vi "Jaccard assignemnts.vi"(9 "cluster centers in":string[](array[string])=["0 -1 1 -4 0 -4 1 -1 0", "0 -1 2 -2 0 -2 2 -1 0", "0 -2 3 -3 0 -3 3 -2 0", "0 -3 4 -4 0 -4 4 -3 0", "0 -1 1 -4 4 -3 0 -3 4 -4 1 -1 0", "0 -1 2 -2 3 -3 0 -3 3 -2 2 -1 0", "0 -4 1 -1 2 -2 0 -2 2 -1 1 -4 0", "0 -4 4 -3 3 -2 0 -2 3 -3 4 -4 0", "0 -1 1 -4 0 -2 3 -3 0 -3 3 -2 0 -4 1 -1 0", "0 -1 2 -2 0 -4 4 -3 0 -3 4 -4 0 -2 2 -1 0"], 11 "patterns in":string[](array[string])) -> (0 "distance values out enhanced multiset)":dbl[][](array[numeric]), 1 "distance values out (multiset)":dbl[][](array[numeric]), 2 "distance values out enhanced (set)":dbl[][](array[numeric]), 3 "distance values out (set)":dbl[][](array[numeric]))   [LabVIEW 2014]
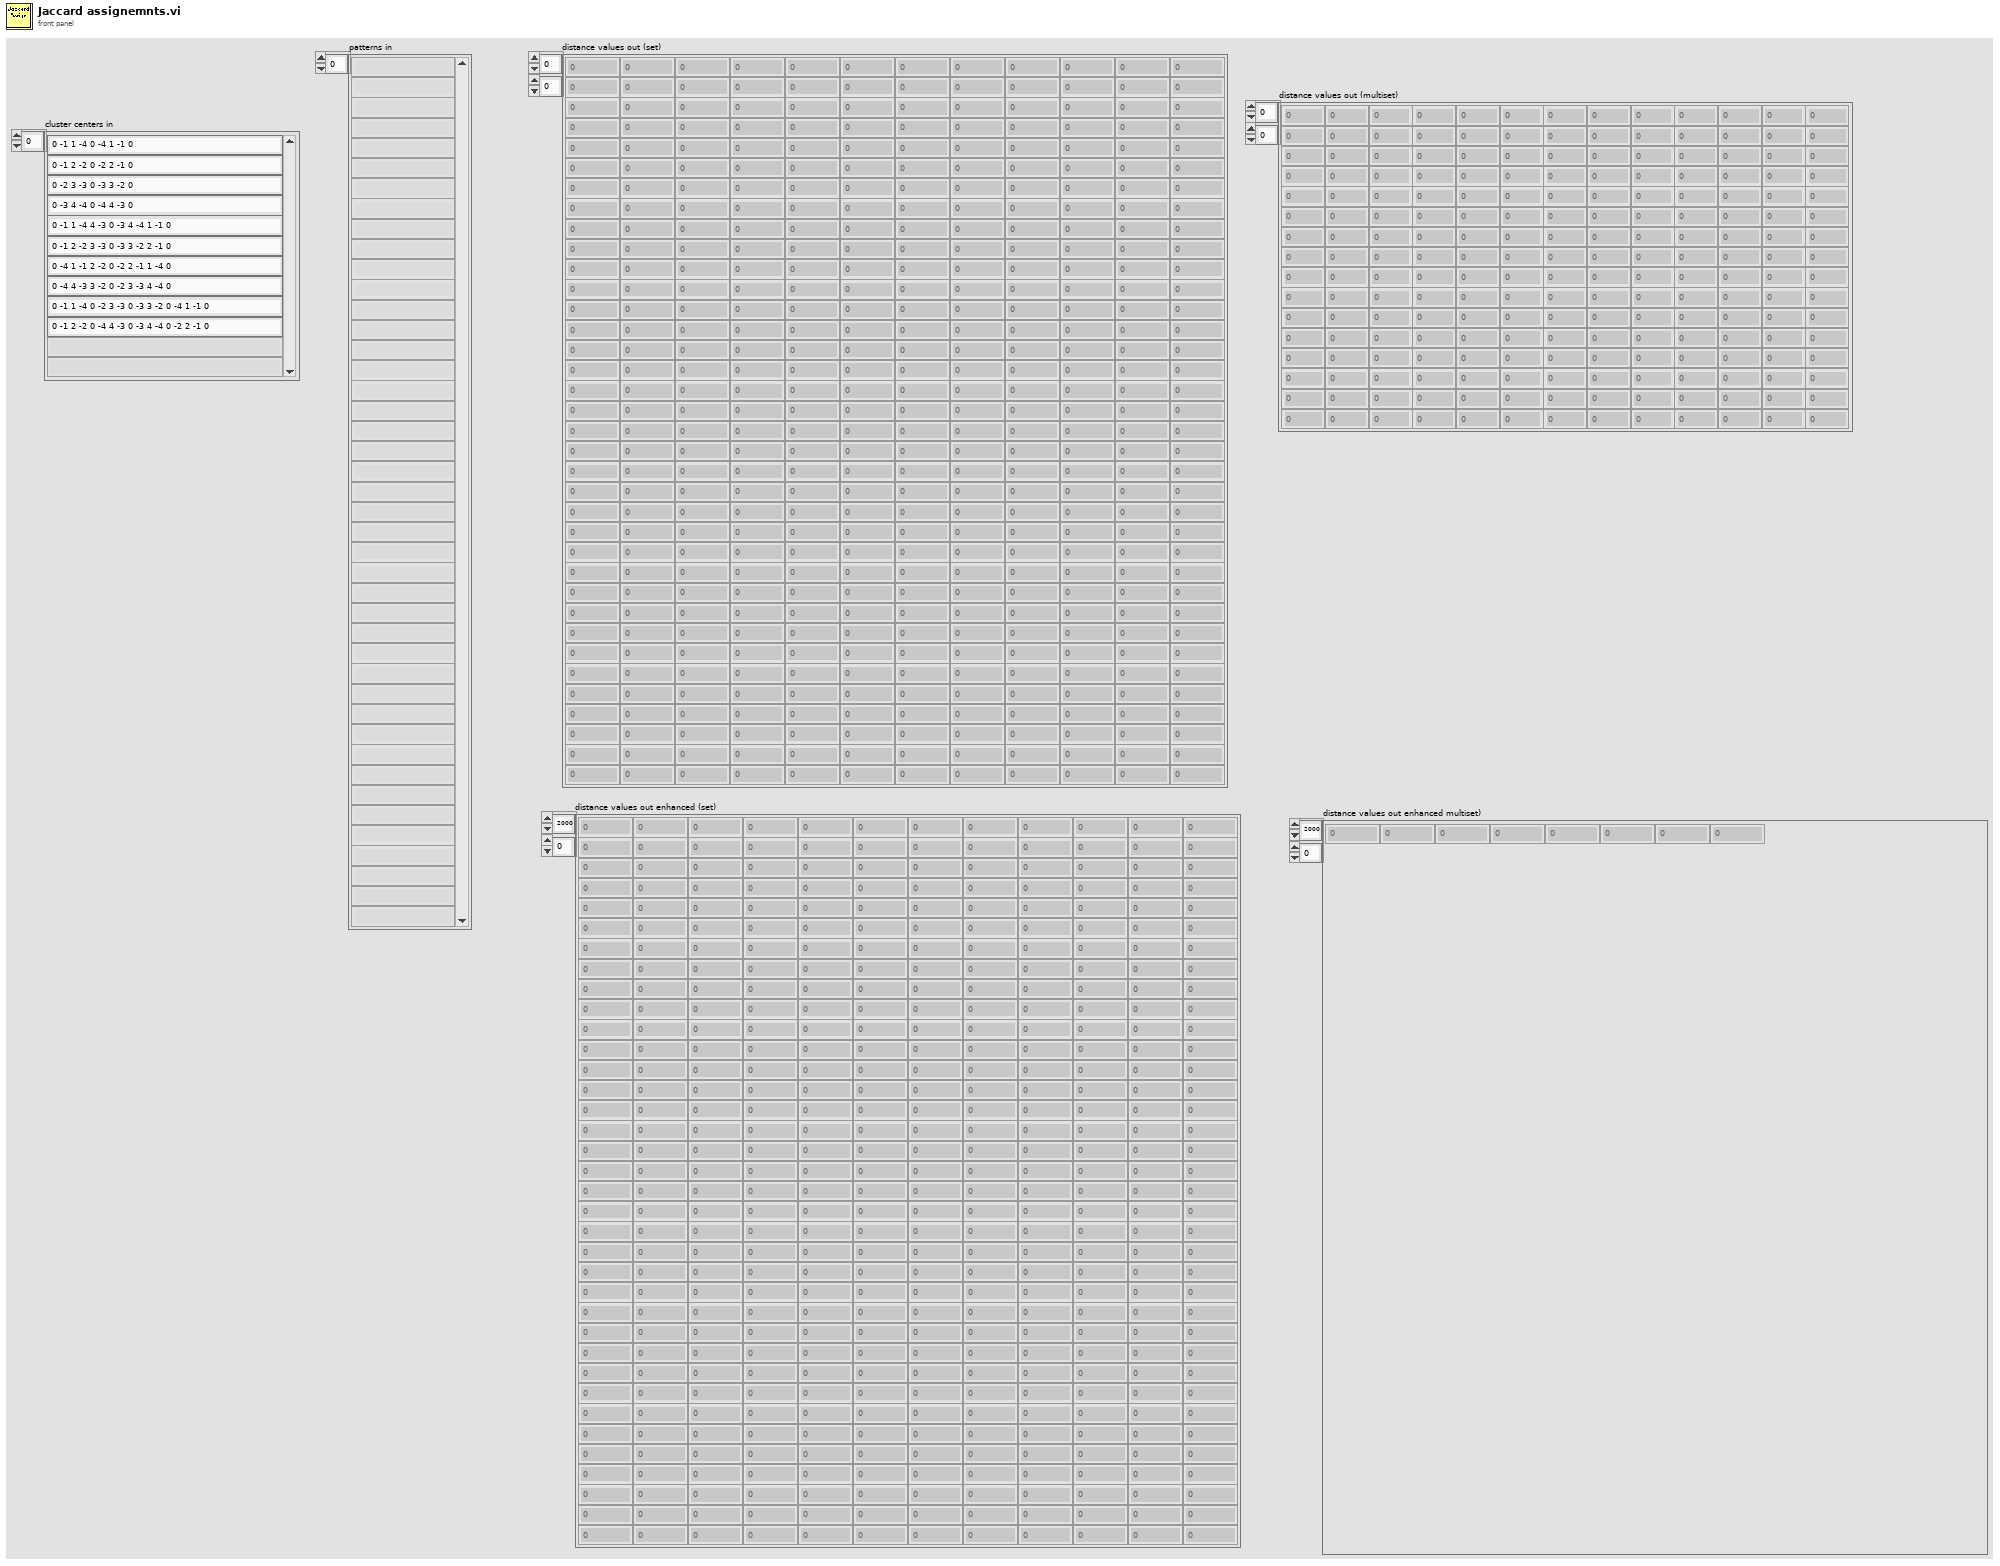
[diagram p1: front panel]
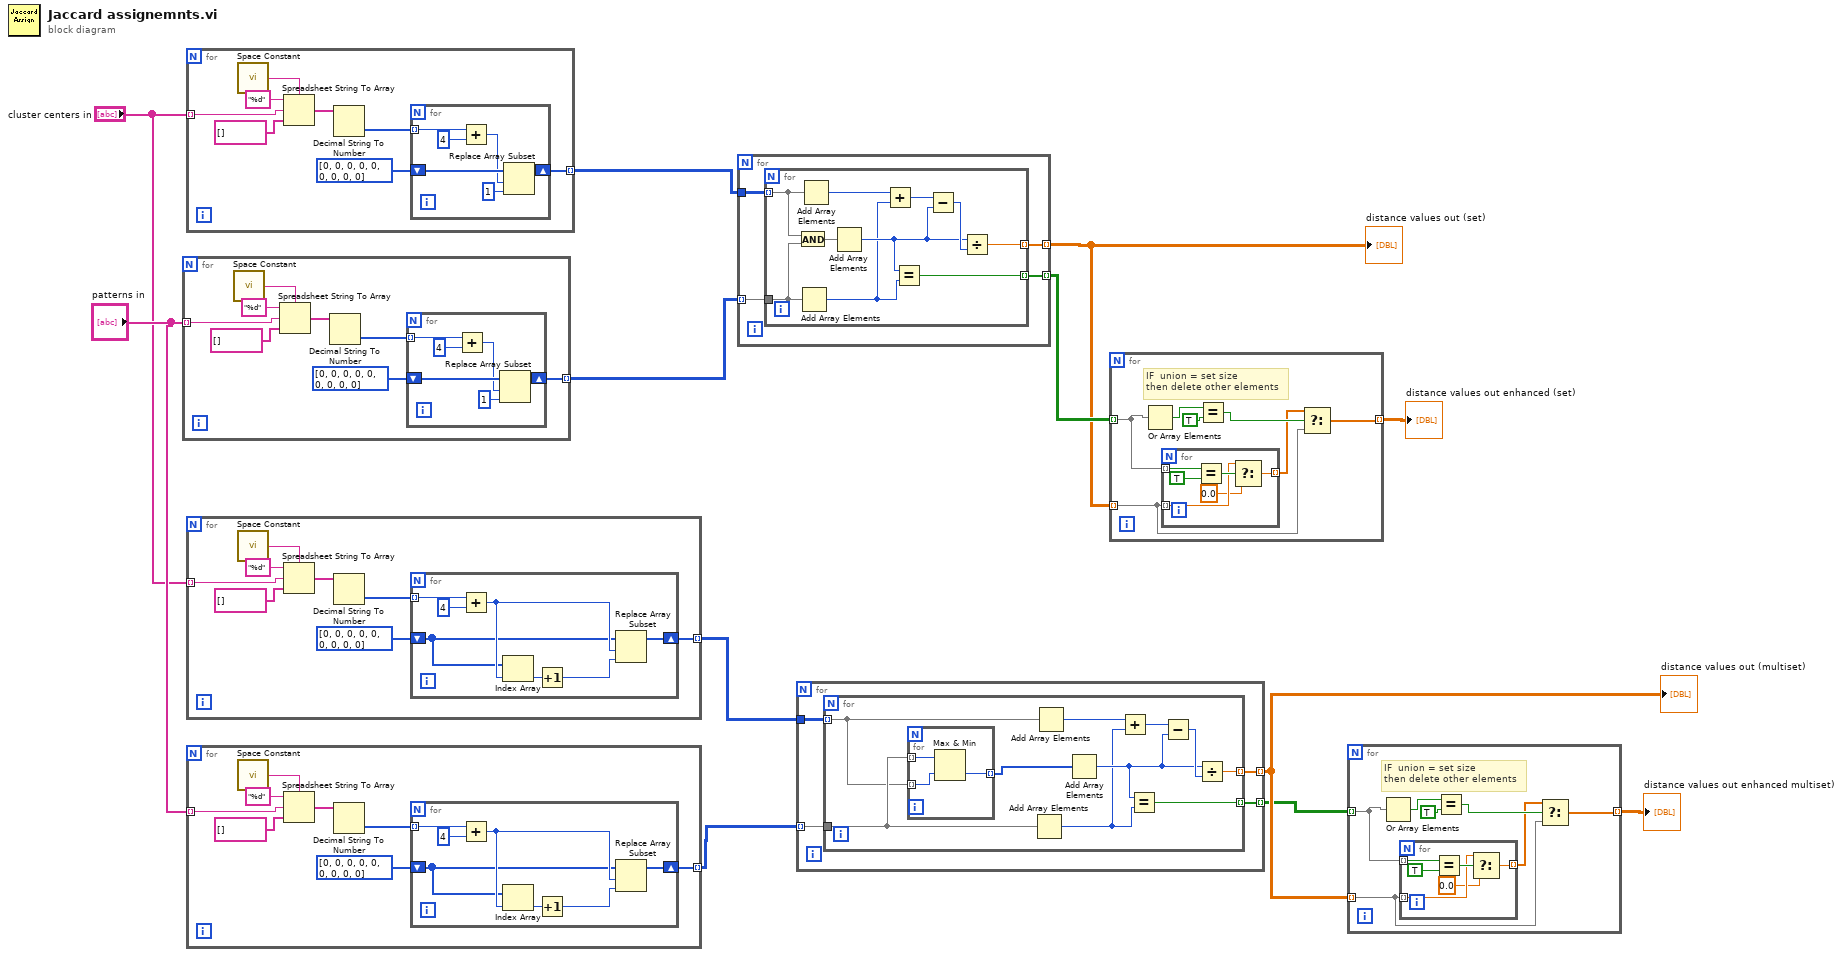
[diagram p0: block diagram]
diagram:
  n1 = for {
    tunnel: "patterns in" -> [w16] mode=indexing
    tunnel: [w13] -> w11 mode=indexing
    n2 = call <vilib>:"Space Constant.vi"() -> ("String"=w17:string)
    n3 = Spreadsheet String To Array(delimiter (Tab)=w17, format string="%d", spreadsheet string=w16, array type (2D Dbl)=string[] []) -> (array=w20:string[])
    n4 = Decimal String To Number(string=w20) -> (number=w15:i32[])  [unwired: 2 in, 1 out]
    n5 = for {
      tunnel: w15 -> [w26] mode=indexing
      shift-right: [w21] -> w13
      shift-left: i32[] [0, 0, 0, 0, 0, 0, 0, 0, 0] ("deleted portion") -> [w24]
      n6 = Add(x=w26, y=4) -> (x+y=w22:i32)
      n7 = Replace Array Subset(array=w24, new element=1 ("new element/subarray"), index=w22) -> (w21:i32[])
    }
  }
  n8 = for {
    tunnel: "cluster centers in" -> [w30] mode=indexing
    tunnel: [w27] -> w12 mode=indexing
    n9 = call <vilib>:"Space Constant.vi"() -> ("String"=w31:string)
    n10 = Spreadsheet String To Array(delimiter (Tab)=w31, format string="%d", spreadsheet string=w30, array type (2D Dbl)=string[] []) -> (array=w34:string[])
    n11 = Decimal String To Number(string=w34) -> (number=w29:i32[])  [unwired: 2 in, 1 out]
    n12 = for {
      tunnel: w29 -> [w40] mode=indexing
      shift-right: [w35] -> w27
      shift-left: i32[] [0, 0, 0, 0, 0, 0, 0, 0, 0] ("deleted portion") -> [w38]
      n13 = Add(x=w40, y=4) -> (x+y=w36:i32)
      n14 = Replace Array Subset(array=w38, new element=1 ("new element/subarray"), index=w36) -> (w35:i32[])
    }
  }
  n15 = for {
    tunnel: "cluster centers in" -> [w44] mode=indexing
    tunnel: [w41] -> w6 mode=indexing
    n16 = call <vilib>:"Space Constant.vi"() -> ("String"=w45:string)
    n17 = Spreadsheet String To Array(delimiter (Tab)=w45, format string="%d", spreadsheet string=w44, array type (2D Dbl)=string[] []) -> (array=w48:string[])
    n18 = Decimal String To Number(string=w48) -> (number=w43:i32[])  [unwired: 2 in, 1 out]
    n19 = for {
      tunnel: w43 -> [w55] mode=indexing
      shift-right: [w53] -> w41
      shift-left: i32[] [0, 0, 0, 0, 0, 0, 0, 0, 0] ("deleted portion") -> [w49]
      n20 = Add(x=w55, y=4) -> (x+y=w52:i32)
      n21 = Index Array(array=w49, index=w52) -> (element=w51:i32)
      n22 = Increment(x=w51) -> (x+1=w50:i32)
      n23 = Replace Array Subset(array=w49, new element=w50, index=w52) -> (w53:i32[])
    }
  }
  n24 = for {
    tunnel: "patterns in" -> [w59] mode=indexing
    tunnel: [w56] -> w5 mode=indexing
    n25 = call <vilib>:"Space Constant.vi"() -> ("String"=w60:string)
    n26 = Spreadsheet String To Array(delimiter (Tab)=w60, format string="%d", spreadsheet string=w59, array type (2D Dbl)=string[] []) -> (array=w63:string[])
    n27 = Decimal String To Number(string=w63) -> (number=w58:i32[])  [unwired: 2 in, 1 out]
    n28 = for {
      tunnel: w58 -> [w70] mode=indexing
      shift-right: [w68] -> w56
      shift-left: i32[] [0, 0, 0, 0, 0, 0, 0, 0, 0] ("deleted portion") -> [w64]
      n29 = Add(x=w70, y=4) -> (x+y=w67:i32)
      n30 = Index Array(array=w64, index=w67) -> (element=w66:i32)
      n31 = Increment(x=w66) -> (x+1=w65:i32)
      n32 = Replace Array Subset(array=w64, new element=w65, index=w67) -> (w68:i32[])
    }
  }
  n33 = for {
    tunnel: w12 -> [w74]
    tunnel: w11 -> [w73] mode=indexing
    tunnel: [w72] -> w8 mode=indexing
    tunnel: [w71] -> w10 mode=indexing
    n34 = for {
      tunnel: w74 -> [w83] mode=indexing
      tunnel: w73 -> [w84]
      tunnel: [w80] -> w72 mode=indexing
      tunnel: [w78] -> w71 mode=indexing
      n35 = And(x=w83, y=w84) -> (x .and. y?=w82:i32[])
      n36 = Add Array Elements(numeric array=w84) -> (sum=w76:i32)
      n37 = Add Array Elements(numeric array=w83) -> (sum=w75:i32)
      n38 = Add Array Elements(numeric array=w82) -> (sum=w77:i32)
      n39 = Add(x=w75, y=w76) -> (x+y=w81:i32)
      n40 = Equal?(x=w77, y=w76) -> (x = y?=w78:bool)
      n41 = Subtract(x=w81, y=w77) -> (x-y=w79:i32)
      n42 = Divide(x=w77, y=w79) -> (x/y=w80:dbl)
    }
  }
  "distance values out (set)" <- w8
  n43 = for {
    tunnel: w6 -> [w88]
    tunnel: w5 -> [w87] mode=indexing
    tunnel: [w86] -> w2 mode=indexing
    tunnel: [w85] -> w1 mode=indexing
    n44 = for {
      tunnel: w88 -> [w90] mode=indexing
      tunnel: w87 -> [w91]
      tunnel: [w97] -> w86 mode=indexing
      tunnel: [w95] -> w85 mode=indexing
      n45 = for {
        tunnel: w91 -> [w101] mode=indexing
        tunnel: w90 -> [w100] mode=indexing
        tunnel: [w99] -> w89 mode=indexing
        n46 = Max & Min(x=w101, y=w100) -> (min(x,y)=w99:i32)  [unwired: 1 out]
      }
      n47 = Add Array Elements(numeric array=w91) -> (sum=w93:i32)
      n48 = Add Array Elements(numeric array=w90) -> (sum=w92:i32)
      n49 = Add Array Elements(numeric array=w89) -> (sum=w94:i32)
      n50 = Add(x=w92, y=w93) -> (x+y=w98:i32)
      n51 = Equal?(x=w94, y=w93) -> (x = y?=w95:bool)
      n52 = Subtract(x=w98, y=w94) -> (x-y=w96:i32)
      n53 = Divide(x=w94, y=w96) -> (x/y=w97:dbl)
    }
  }
  "distance values out (multiset)" <- w2
  n54 = for {
    tunnel: w10 -> [w105] mode=indexing
    tunnel: [w107] -> w9 mode=indexing
    tunnel: w8 -> [w102] mode=indexing
    # "IF  union = set size \nthen delete other elements"
    n55 = Or Array Elements(Boolean array=w105) -> (logical OR=w104:bool)
    n56 = for {
      tunnel: w105 -> [w112] mode=indexing
      tunnel: [w113] -> w106 mode=indexing
      tunnel: w102 -> [w110] mode=indexing
      n57 = Equal?(x=w112, y=TRUE) -> (x = y?=w114:bool)
      n58 = Select(t=w110, s=w114, f=0.0) -> (s? t:f=w113:dbl)
    }
    n59 = Equal?(x=w104, y=TRUE) -> (x = y?=w108:bool)
    n60 = Select(t=w106, s=w108, f=w102) -> (s? t:f=w107:dbl[])
  }
  "distance values out enhanced (set)" <- w9
  n61 = for {
    tunnel: w1 -> [w118] mode=indexing
    tunnel: [w120] -> w3 mode=indexing
    tunnel: w2 -> [w115] mode=indexing
    # "IF  union = set size \nthen delete other elements"
    n62 = Or Array Elements(Boolean array=w118) -> (logical OR=w117:bool)
    n63 = for {
      tunnel: w118 -> [w125] mode=indexing
      tunnel: [w126] -> w119 mode=indexing
      tunnel: w115 -> [w123] mode=indexing
      n64 = Equal?(x=w125, y=TRUE) -> (x = y?=w127:bool)
      n65 = Select(t=w123, s=w127, f=0.0) -> (s? t:f=w126:dbl)
    }
    n66 = Equal?(x=w117, y=TRUE) -> (x = y?=w121:bool)
    n67 = Select(t=w119, s=w121, f=w115) -> (s? t:f=w120:dbl[])
  }
  "distance values out enhanced multiset)" <- w3
